vi "Set IInstrument.vi"(8 "error in":errorcluster, 10 "IInstrument":refnum<class "IInstrument.lvclass">, 11 "IVirtual Instrument in":refnum<class "IVirtual Instrument.lvclass">) -> (0 "error out":errorcluster, 3 "IVirtual Instrument out":refnum<class "IVirtual Instrument.lvclass">)   [LabVIEW 2019, in "IVirtual Instrument.lvclass"]
uses:
  IVirtual Instrument.lvclass
  IInstrument/IInstrument.lvclass
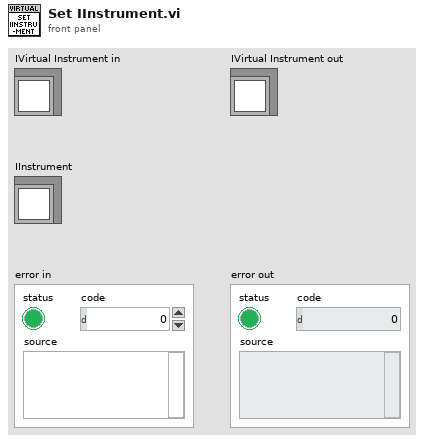
[diagram p1: front panel]
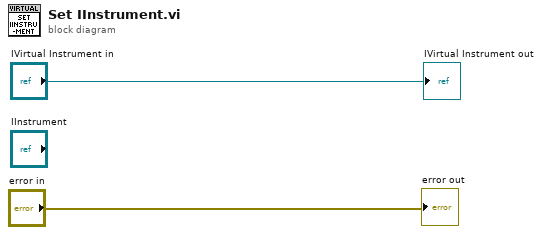
[diagram p0: block diagram]
diagram:
  "IVirtual Instrument out" <- "IVirtual Instrument in"
  "error out" <- "error in"
